vi "PH_DeformableMirror.contents.vi"   [LabVIEW 2014, in "PH_DeformableMirror.lvlib"]
uses:
  PH_DeformableMirror.lvlib
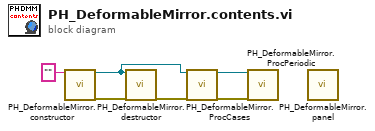
[diagram p0: block diagram]
diagram:
  n1 = call "PH_DeformableMirror.constructor.vi"("name"="") -> ("i ref out"=w1:refnum<vi>, "error out"=w5:errorcluster)  [unwired: 16 in, 1 out]
  n2 = call "PH_DeformableMirror.destructor.vi"("i ref in"=w1, "error in(no error)"=w5) -> ("error out"=w4:errorcluster)  [unwired: 17 in]
  n3 = call "PH_DeformableMirror.ProcCases.vi"("i ref in"=w1, "error in (no error)"=w4) -> ("i ref out"=w3:refnum<vi>, "error out"=w2:errorcluster)  [unwired: 15 in, 1 out]
  n4 = call "PH_DeformableMirror.ProcPeriodic.vi"("i ref in"=w3, "error in (no error)"=w2) -> ()  [unwired: 15 in, 3 out]
  n5 = call "PH_DeformableMirror.panel.vi"() -> ()  [unwired: 19 in, 1 out]
